vi "Drive Path.vi"(6 "Synchronication":enum16{"Start", "Wait"}(ring)=enum."Wait", 7 "Description":string, 8 "Command Info In":T2, 11 "Path":T1={"Path"=[], "MaxVel"=0.0, "MaxAccel"=0.0, "Backwards?"=FALSE, "PointSpacing"=0.0, "LookaheadDist"=0.0, "Speed/Curve"=1.8, "SlowDistanceAtEnd"=12.0, "SlowSpeed"=15.0} {"SlowSpeed" format="%#_13g"; "SlowDistanceAtEnd" format="%#_13g"; "Speed/Curve" format="%#_13g"}) -> (0 "Command Info Out":T2)   [LabVIEW 2017]
doc: "This VI notifies the subsystem to perform this command for the given duration, then go back to the default state. Synchronization determines whether this VI Starts the operation and returns immediately, or waits for the operation to complete. The first option is commonly used for TeleOp, and the second for Autonomous sequencing."
uses:
  <vilib>/Rock Robotics/WPI/Framework/Command Status Info.ctl
  <vilib>/Rock Robotics/WPI/Framework/Completion Status.ctl
  <vilib>/Rock Robotics/WPI/Framework/Completion Notifier.ctl
  Shared/RobotNeededPathData.ctl
  Implementation/Drive Setpoints.ctl
  Implementation/Drive Operations.ctl
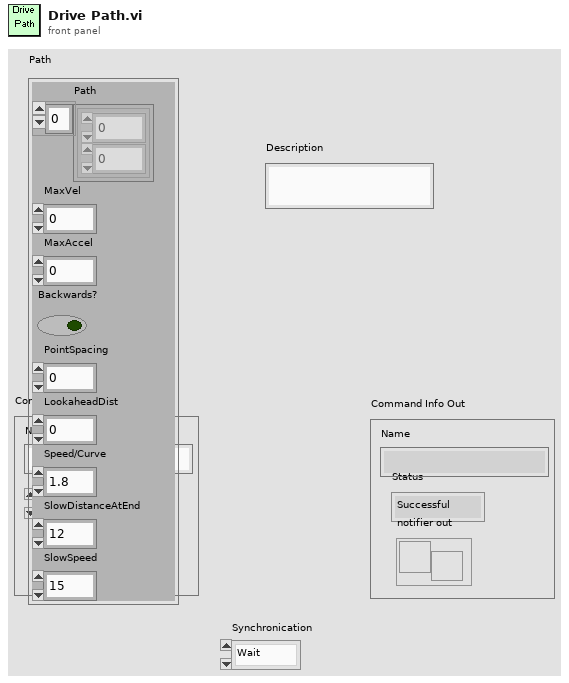
[diagram p1: front panel]
types:
  T1 = typedef "RobotNeededPathData.ctl" = cluster{"Path":cluster{dbl, dbl}[], "MaxVel":dbl, "MaxAccel":dbl, "Backwards?":bool, "PointSpacing":dbl, "LookaheadDist":dbl, "Speed/Curve":dbl, "SlowDistanceAtEnd":dbl, "SlowSpeed":dbl}
  T2 = typedef "Command Status Info.ctl" = cluster{"Name":string, "Status":T3, "notifier out":T4}
  T3 = typedef "Completion Status.ctl" = enum16{"Successful", "Aborted", "Incomplete"}
  T4 = typedef "Completion Notifier.ctl" = refnum<notifier>
  T5 = typedef "Drive Setpoints.ctl" = cluster{"Operation":T6, "Left Speed":dbl, "Right Speed":dbl, "Duration":dbl, "Speed":dbl, "Start Angle":dbl, "Target Angle":dbl, "Distance (inch)":dbl, "Start Point (inch)":dbl, "RobotNeededPathData":T1}
  T6 = typedef "Drive Operations.ctl" = enum16{"Reserve", "Read Current", "Immediate", "Drive for Time", "Drive for Distance", "Turn to Angle", "Arc Turn", "Drive Path"}
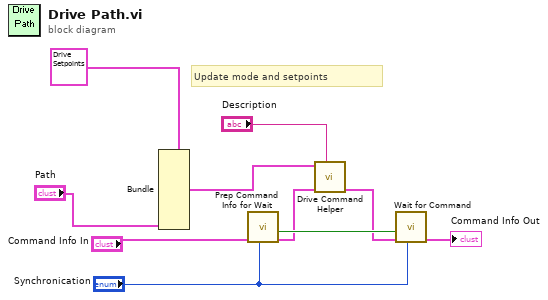
[diagram p0: block diagram]
diagram:
  # "Update mode and setpoints"
  n1 = Bundle(cluster=T5 {"Operation"=enum."Drive Path", "Left Speed"=0.0, "Right Speed"=0.0, "Duration"=0.0, "Speed"=0.0, "Start Angle"=0.0, "Target Angle"=0.0, "Distance (inch)"=0.0, "Start Point (inch)"=0.0, "RobotNeededPathData"={"Path"=[], "MaxVel"=0.0, "MaxAccel"=0.0, "Backwards?"=FALSE, "PointSpacing"=0.0, "LookaheadDist"=0.0, "Speed/Curve"=1.8, "SlowDistanceAtEnd"=12.0, "SlowSpeed"=15.0}} ("SubSystem Data"), "RobotNeededPathData"="Path") -> (w3:T5)  [unwired: 9 in]
  n2 = call <vilib>:"Prep Command Info for Wait.vi"("Synchronication"="Synchronication", "Command Info"="Command Info In") -> ("Command Info"=w7:T2, "Allocated"=w8:bool)  [unwired: 8 in]
  n3 = call "Drive Command Helper.vi"("Description"="Description", "Command Info In"=w7, "SubSystem Data"=w3) -> ("Command Info Out"=w4:T2)  [unwired: 6 in, 2 out]
  n4 = call <vilib>:"Wait for Command.vi"("Synchronication"="Synchronication", "Command Info in"=w4, "Allocated"=w8) -> ("Command Info out"=→"Command Info Out":T2)  [unwired: 8 in]
